vi "SetTransVol.vi"(8 "错误输入（无错误）":errorcluster, 10 "发射电压":u32) -> (0 "错误输出":errorcluster)   [LabVIEW 2018]
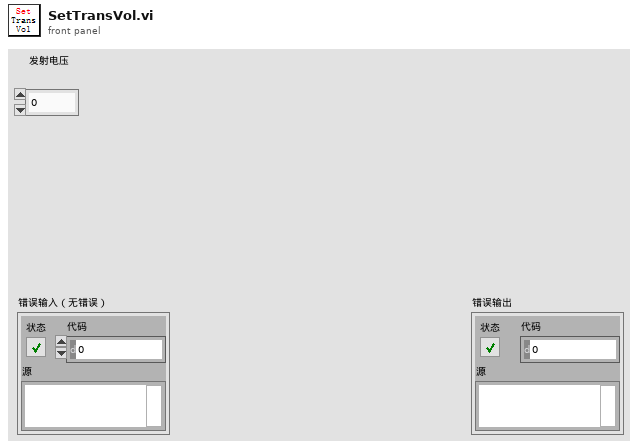
[diagram p1: front panel]
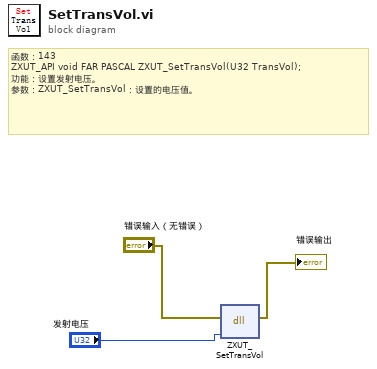
[diagram p0: block diagram]
diagram:
  # "函数：143\nZXUT_API void\tFAR PASCAL ZXUT_SetTransVol(U32 TransVol);\n功能：设置发射电压。\n参数：ZXUT_SetTransVol：设置的电压值。"
  n1 = dll-call lib="PTH2Rabs E软件项目超声超声子VI函数VI\tTCG处理ZXUTConfigMgr.dll" fn="ZXUT_SetTransVol"(error in="错误输入（无错误）", "TransVol"="发射电压") -> (error out=→"错误输出":errorcluster)  [unwired: 4 in, 1 out]
